vi "getFractionJulianDate.vi"() -> (0 "Fraction of the day":dbl format="%#_13g")   [LabVIEW 2015]
panel:
  out "Number of seconds \nsince 1904":dbl format="%#_13g"
  out "Number of seconds between\n1904 and today 00:00":dbl format="%#_13g"
  out "This day at 00:00":timestamp
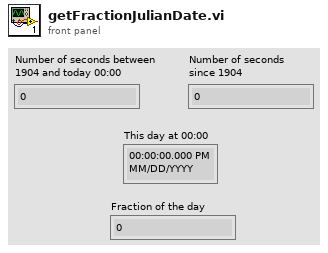
[diagram p1: front panel]
types:
  T1 = cluster{dbl, i32, i32, i32, i32, i32, i32, i32, i32, i32}
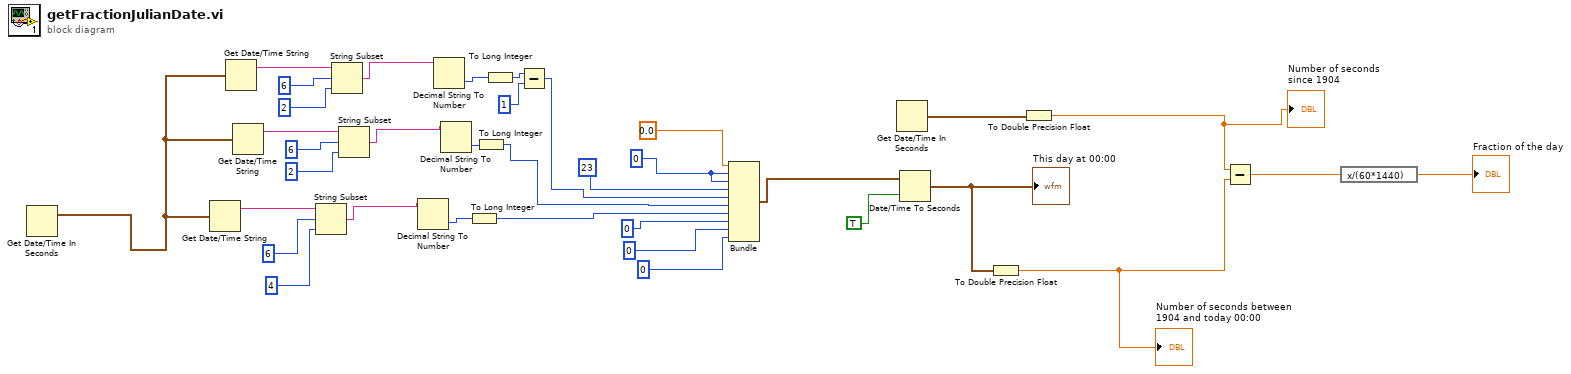
[diagram p0: block diagram]
diagram:
  w17 = 0
  (unwired) 6
  (unwired) 6
  (unwired) 6
  n1 = Get Date/Time In Seconds() -> (seconds since 1Jan1904=w1:timestamp)
  n2 = Get Date/Time String(seconds (now)=w1) -> (date string=w35:string)  [unwired: 2 in, 1 out]
  n3 = Get Date/Time String(seconds (now)=w1) -> (date string=w3:string)  [unwired: 2 in, 1 out]
  n4 = Get Date/Time String(seconds (now)=w1) -> (date string=w16:string)  [unwired: 2 in, 1 out]
  n5 = String Subset(string=w35, offset (0)=6, length (rest)=4) -> (substring=w27:string)
  n6 = String Subset(string=w3, offset (0)=0, length (rest)=2) -> (substring=w2:string)
  n7 = String Subset(string=w16, offset (0)=3, length (rest)=2) -> (substring=w19:string)
  n8 = Decimal String To Number(string=w27) -> (number=w26:i32)  [unwired: 2 in, 1 out]
  n9 = Decimal String To Number(string=w2) -> (number=w22:i32)  [unwired: 2 in, 1 out]
  n10 = Decimal String To Number(string=w19) -> (number=w18:i32)  [unwired: 2 in, 1 out]
  n11 = To Long Integer(number=w26) -> (32bit integer=w6:i32)
  n12 = To Long Integer(number=w18) -> (32bit integer=w7:i32)
  n13 = To Long Integer(number=w22) -> (32bit integer=w14:i32)
  n14 = Subtract(x=w14, y=1) -> (x-y=w13:i32)
  n15 = Bundle(0.0, w17, w17, 23, w13, w7, w6, 0, 0, 0) -> (w15:T1)  [unwired: 1 in]
  n16 = Get Date/Time In Seconds() -> (seconds since 1Jan1904=w11:timestamp)
  n17 = Date/Time To Seconds(1:TRUE, 2:w15) -> (0:w10:timestamp)
  "This day at 00:00" <- w10
  n18 = To Double Precision Float(number=w10) -> (double precision float=w9:dbl)
  "Number of seconds between\n1904 and today 00:00" <- w9
  n19 = To Double Precision Float(number=w11) -> (double precision float=w8:dbl)
  "Number of seconds \nsince 1904" <- w8
  n20 = Subtract(x=w8, y=w9) -> (x-y=w5:dbl)
  n21 = expression code="x/(60*1440)"(w5) -> (→"Fraction of the day":dbl)
